vi "Read Raw Result.vi"(8 "error in (no error)":errorcluster, 11 "ReadCommand in":refnum<class "ReadCommand.lvclass">) -> (0 "error out":errorcluster, 2 "Raw Result":string, 3 "ReadCommand out":refnum<class "ReadCommand.lvclass">)   [LabVIEW 2023, in "HAF.lvlib" / "ReadCommand.lvclass"]
doc: "Returns the Raw Result value."
uses:
  ReadCommand.lvclass
  ReadCommand.lvclass/ReadCommand.ctl
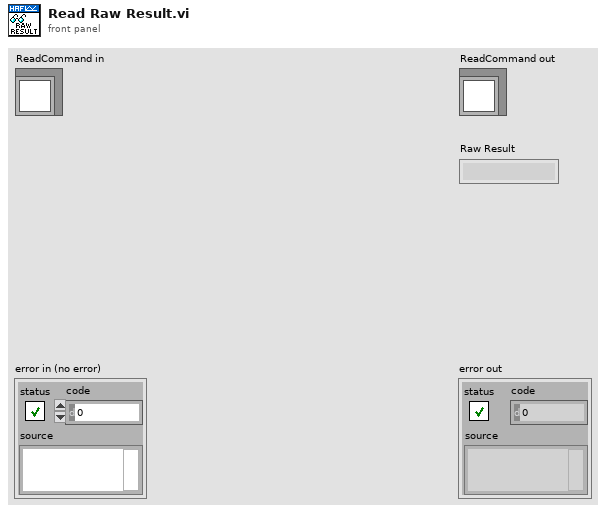
[diagram p1: front panel]
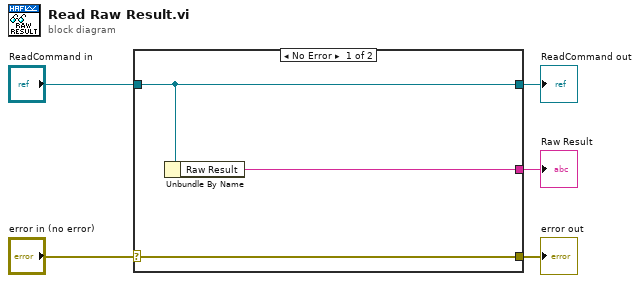
[diagram p0: block diagram]
diagram:
  n1 = case shown="No Error" "error in (no error)" {
    selector: "error in (no error)" -> [w8 w9]
    tunnel: [w8 w9] -> w4
    tunnel: [w7 w10] -> w2
    tunnel: "ReadCommand in" -> [w7 w10]
    tunnel: [w6 _] -> w1
    frame No Error {
      n2 = Unbundle By Name(w7) -> ("Raw Result"=w6:string)
    }
    frame Error {
    }
  }
  "error out" <- w4
  "ReadCommand out" <- w2
  "Raw Result" <- w1
